vi "configure.vi"(8 "error in (no error)":errorcluster, 9 "Value":i32, 10 "ILC":refnum<class "ILC.lvclass">, 11 "ConfigureILCDIStrategy in":refnum<class "ConfigureILCDIStrategy.lvclass">) -> (0 "error out":errorcluster, 2 "ILC 2":refnum<class "ILC.lvclass">, 3 "ConfigureILCDIStrategy out":refnum<class "ConfigureILCDIStrategy.lvclass">)   [LabVIEW 2015, in "ConfigureILCDIStrategy.lvclass"]
uses:
  ConfigureILCDIStrategy/ConfigureILCDIStrategy.lvclass
  <userlib>/Common/ILC/ILC/ILC.lvclass
  ConfigureILCDIStrategy/ConfigureILCDIStrategy.lvclass/ConfigureILCDIStrategy.ctl
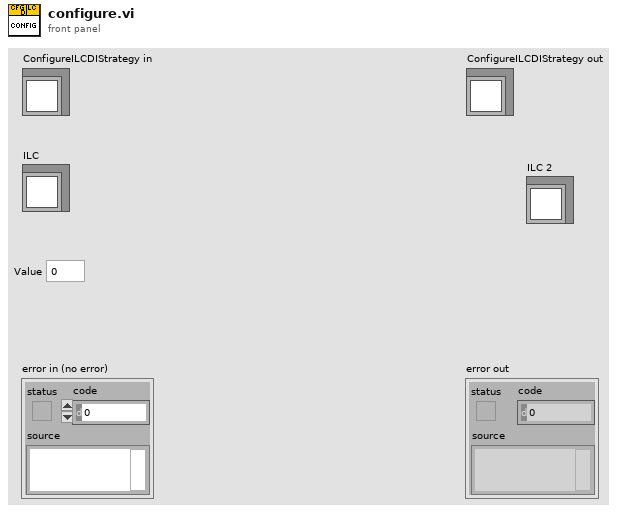
[diagram p1: front panel]
types:
  T1 = typedef "ILCBTTypedefs.lvlib/Digital Signal Level.ctl" = enum16{"Low", "High"}
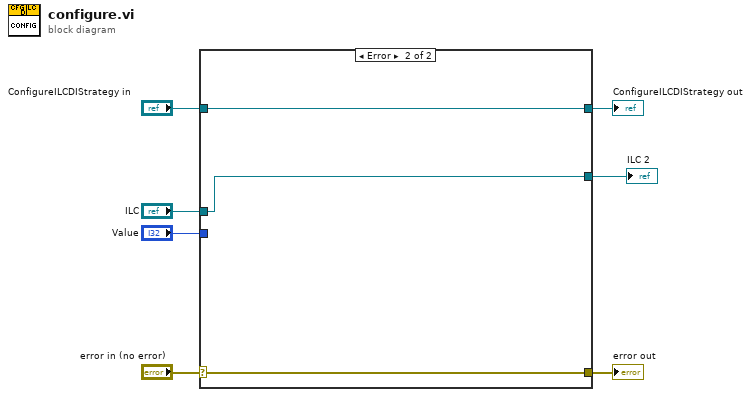
[diagram p0: block diagram]
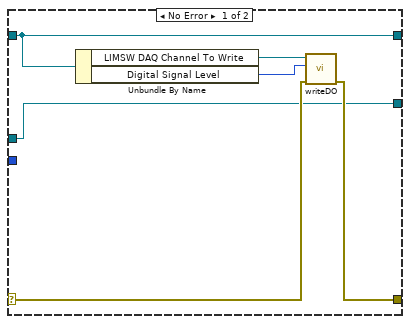
[diagram p2: hidden frame]
diagram:
  n1 = case shown="Error" "error in (no error)" {
    selector: "error in (no error)" -> [w10 w16]
    tunnel: [w9 w16] -> w6
    tunnel: [w12 w15] -> w4
    tunnel: "ConfigureILCDIStrategy in" -> [w12 w15]
    tunnel: "ILC" -> [w8 w14]
    tunnel: "Value" -> [_ _]
    tunnel: [w8 w14] -> w1
    frame No Error {
      n2 = Unbundle By Name(w12) -> ("LIMSW DAQ Channel To Write"=w11:refnum<k21>, "Digital Signal Level"=w13:T1)
      n3 = call "writeDO.vi"("error in"=w10, "Digital Signal Level"=w13, "DAQmx Global Channel"=w11) -> ("error out"=w9:errorcluster)  [unwired: 8 in]
    }
    frame Error {
    }
  }
  "error out" <- w6
  "ConfigureILCDIStrategy out" <- w4
  "ILC 2" <- w1
